vi "FT_Write_EEPROM_User_Area.vi"(1 "User Area Data In":u8[](array[numeric]) format="%x", 2 "Handle":u64) -> (0 "FT_Status":u32(ring) items=["FT_OK", "FT_INVALID_HANDLE", "FT_DEVICE_NOT_FOUND", "FT_DEVICE_NOT_OPENED", "FT_IO_ERROR", "FT_INSUFFICIENT_RESOURCES", "FT_INVALID_PARAMETER", "FT_INVALID_BAUD_RATE", "FT_DEVICE_NOT_OPENED_FOR_ERASE", "FT_DEVICE_NOT_OPENED_FOR_WRITE", "FT_FAILED_TO_WRITE_DEVICE", "FT_EEPROM_READ_FAILED", "FT_EEPROM_WRITE_FAILED", "FT_EEPROM_ERASE_FAILED", "FT_EEPROM_NOT_PRESENT", "FT_EEPROM_NOT_PROGRAMMED", "FT_INVALID_ARGS", "FT_NOT_SUPPORTED", "FT_OTHER_ERROR"])   [LabVIEW 2019, in "D2XX.lvlib"]
uses:
  D2XX.lvlib
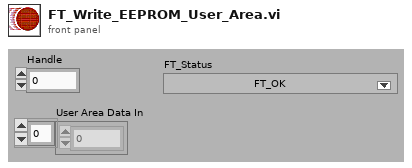
[diagram p1: front panel]
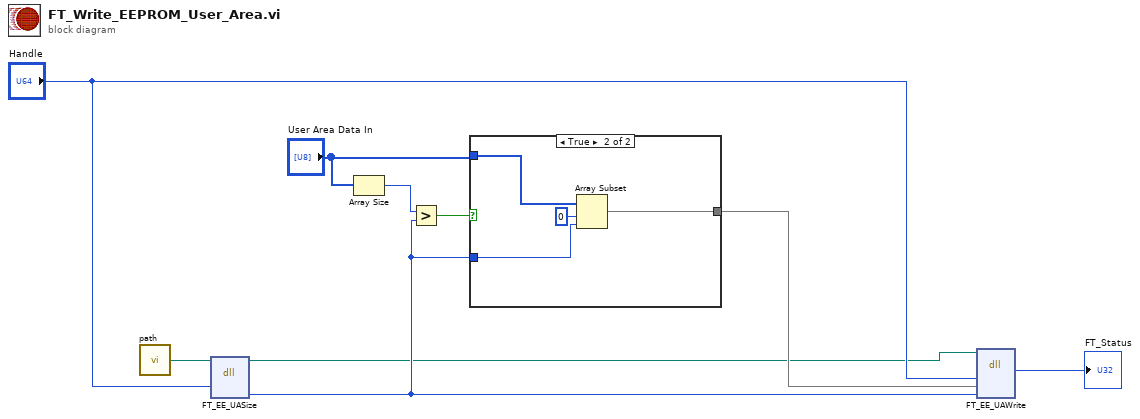
[diagram p0: block diagram]
diagram:
  n1 = call "path.vi"() -> ("lib path"=w5:path)
  n2 = dll-call lib="FTD2XX.dll" fn="FT_EE_UASize"(path in=w5, "Handle"="Handle") -> (path out=w6:path, "UASize"=w8:u32)  [unwired: 5 in, 1 out]
  n3 = Array Size(array="User Area Data In") -> (size(s)=w3:i32)
  n4 = Greater?(x=w3, y=w8) -> (0:w4:bool)
  n5 = case shown="True" w4 {
    tunnel: "User Area Data In" -> [w10 w14]
    tunnel: w8 -> [_ w11]
    tunnel: [w10 w12] -> w7
    frame False {
    }
    frame True {
      n6 = Array Subset(array=w14, index=u16 0, length=w11) -> (w12:u8[])
    }
  }
  n7 = dll-call lib="FTD2XX.dll" fn="FT_EE_UAWrite"(path in=w6, "Handle"="Handle", "Buffer"=w7, "DataLength"=w8) -> (→"FT_Status":u32)  [unwired: 5 in, 2 out]
